vi "Initialize.vi"(8 "error in (no error)":errorcluster, 11 "KNF Settings In":T1={"VISA resource name"="", "Simulated?"=TRUE}) -> (0 "error IO":errorcluster, 1 "Initialized":bool, 2 "No Pump Connected":bool, 3 "KNF Settings Out":T1={"VISA resource name"="", "Simulated?"=TRUE})   [LabVIEW 2018, in "KNF SIMDOS.lvlib"]
uses:
  KNF SIMDOS.lvlib
  Settings Cluster plus SIMDOS.ctl
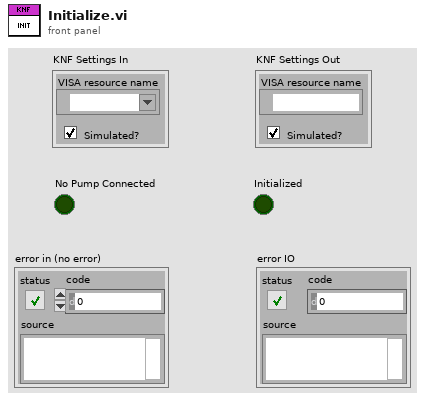
[diagram p1: front panel]
types:
  T1 = typedef "KNF SIMDOS.lvlib/Settings Cluster plus SIMDOS.ctl" = cluster{"VISA resource name":refnum<visa-resource-name>, "Simulated?":bool}
  T2 = cluster{"VISA resource name":refnum<visa-resource-name>, "Simulated?":bool}
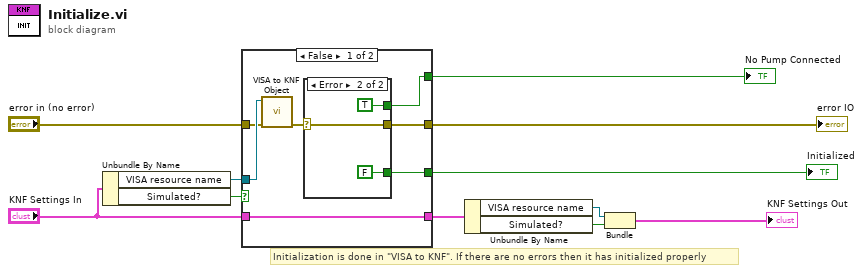
[diagram p0: block diagram]
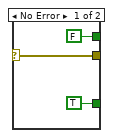
[diagram p2: hidden frame]
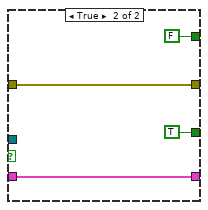
[diagram p3: hidden frame]
diagram:
  # "Initialization is done in \"VISA to KNF\". If there are no errors then it has initialized properly"
  n1 = Unbundle By Name("KNF Settings In") -> ("VISA resource name"=w11:refnum<visa-resource-name>, "Simulated?"=w10:bool)
  n2 = case shown="False" w10 {
    tunnel: w11 -> [w15 _]
    tunnel: [w18 w28] -> w5
    tunnel: "KNF Settings In" -> [w18 w28]
    tunnel: [w17 FALSE] -> w9
    tunnel: "error in (no error)" -> [w14 w26]
    tunnel: [w16 w26] -> w7
    tunnel: [w12 TRUE] -> w1
    frame False {
      n3 = call "VISA to KNF Object.vi"("error in (no error)"=w14, "VISA resource name"=w15) -> ("error out"=w13:errorcluster)  [unwired: 8 in, 1 out]
      n4 = case shown="Error" w13 {
        selector: w13 -> [w20 w23]
        tunnel: [FALSE TRUE] -> w17
        tunnel: [w20 w23] -> w16
        tunnel: [TRUE FALSE] -> w12
        frame No Error {
        }
        frame Error {
        }
      }
    }
    frame True {
    }
  }
  "No Pump Connected" <- w9
  "error IO" <- w7
  "Initialized" <- w1
  n5 = Unbundle By Name(w5) -> ("VISA resource name"=w4:refnum<visa-resource-name>, "Simulated?"=w3:bool)
  n6 = Bundle("VISA resource name"=w4, "Simulated?"=w3) -> (→"KNF Settings Out":T2)  [unwired: 1 in]
